vi "CMC_Addition_or_Subtraction.vi"() -> ()   [LabVIEW 2013]
doc: "This is a sample VI used to demonstrate basic functions on the LabVIEW block diagram."
panel:
  in  "Add/Subtract":bool
  out "Result":dbl
  in  "B":dbl min=0.0 max=100.0 step=1.0
  in  "A":dbl
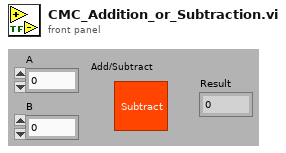
[diagram p1: front panel]
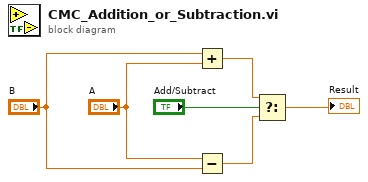
[diagram p0: block diagram]
diagram:
  n1 = Add(x="B", y="A") -> (x+y=w4:dbl)
  n2 = Subtract(x="A", y="B") -> (x-y=w1:dbl)
  n3 = Select(t=w4, s="Add/Subtract", f=w1) -> (s? t:f=→"Result":dbl)
